vi "test1-ProcessSyncMessageInCSMLoop(OnlyReceive).vi"(8 "error in (no error)":errorcluster, 11 "TestCase in":refnum<class "testcase-CSMAddonLoopSupport.lvclass">) -> (0 "error out":errorcluster, 3 "TestCase out":refnum<class "testcase-CSMAddonLoopSupport.lvclass">)   [LabVIEW 2017, in "testcase-CSMAddonLoopSupport.lvclass"]
uses:
  testcase-CSMAddonLoopSupport.lvclass
  4585ddd5-ba69-4fd4-94fe-207595864cbd.vi
  a7620e19-6451-46a1-85ca-ade5edb58587.vi
  55fec5d7-cd22-46f7-b641-2c7c49619fc8.vi
  <vilib>/addons/_JKI Toolkits/VI Tester/TestCase.llb/TestCase.lvclass
  src/user.lib/_NEVSTOP/Communicable State Machine(CSM)/Communicable State Machine.lvlib
  C:/Program Files (x86)/National Instruments/LabVIEW 2017/vi.lib/addons/_JKI Toolkits/VI Tester/TestCase.llb/TestCase.lvclass
panel:
  out "error out2":errorcluster
  out "LoopCount":i32
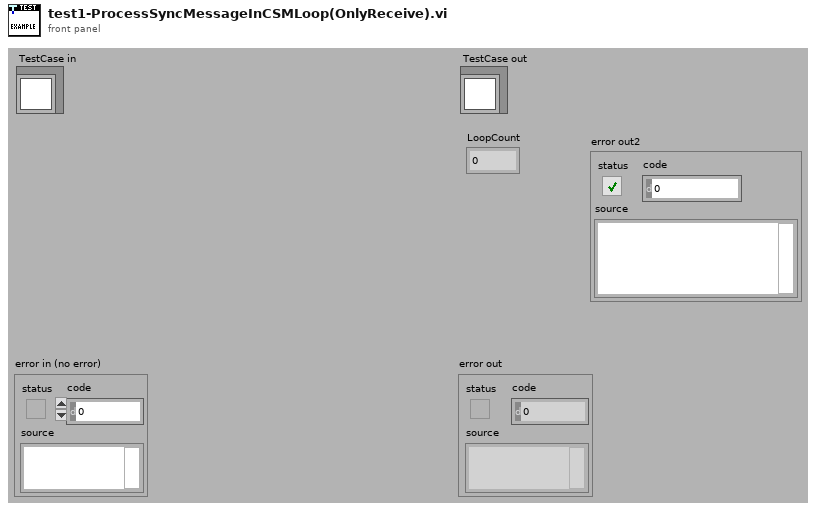
[diagram p1: front panel]
types:
  T1 = cluster{"Arguments":string, "Response":string, "error":errorcluster}
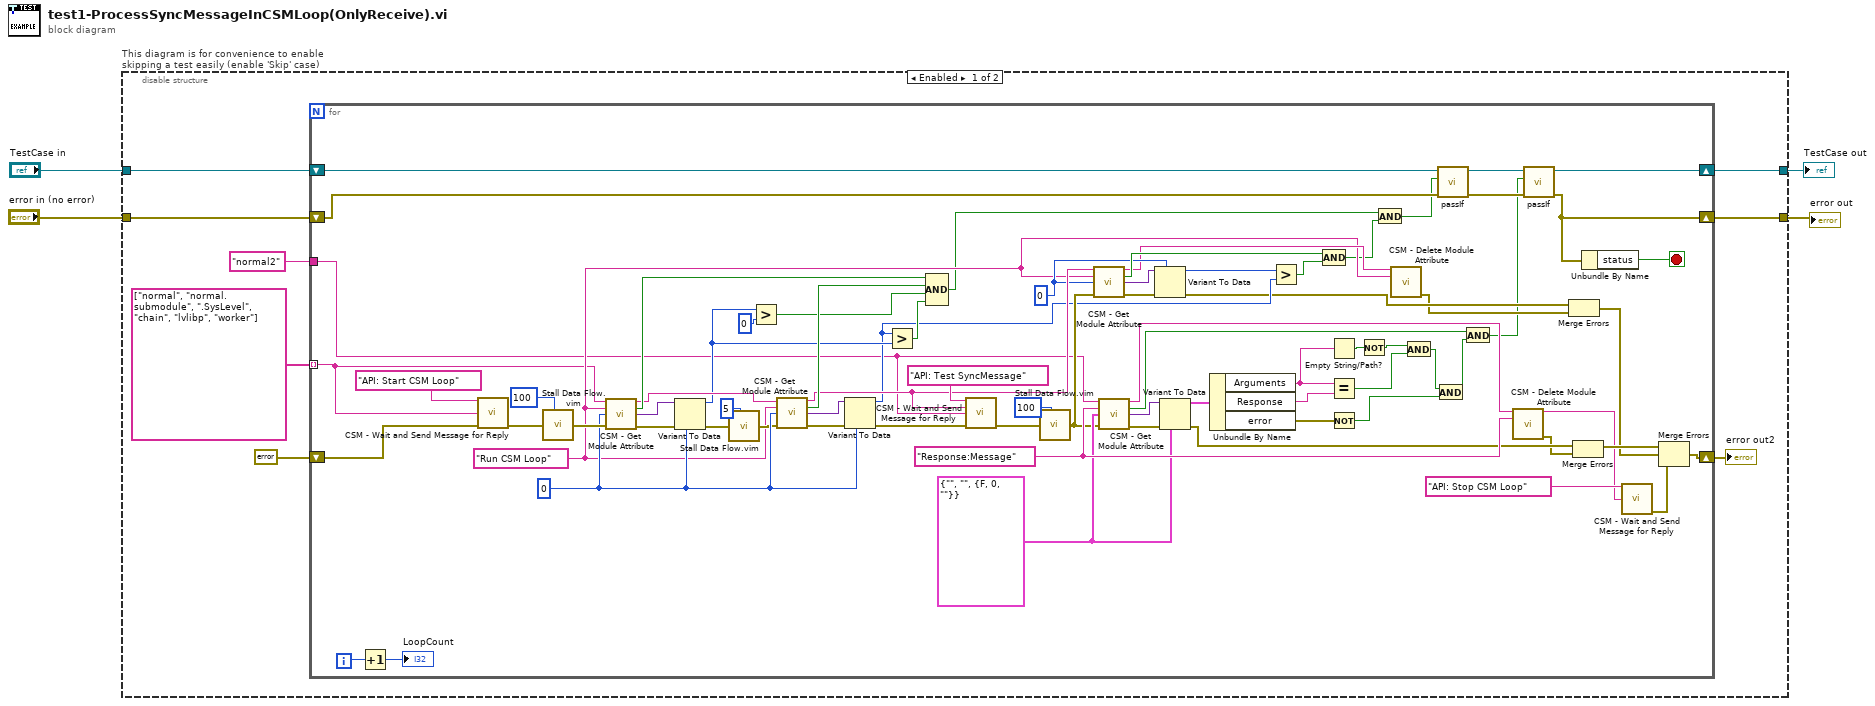
[diagram p0: block diagram]
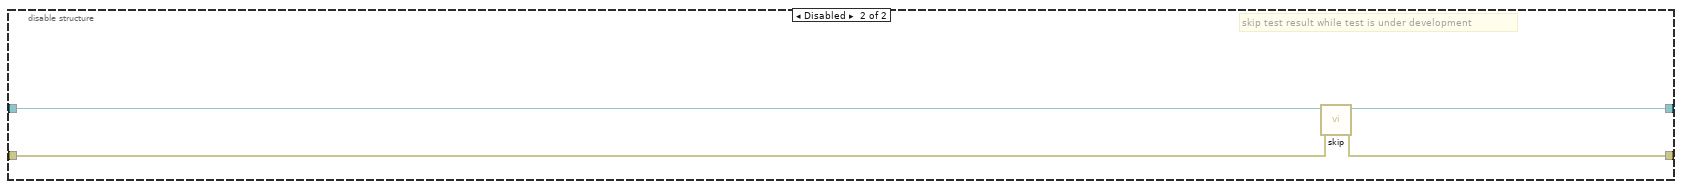
[diagram p2: hidden frame]
diagram:
  n1 = disable-structure "This diagram is for convenience to enable skipping a test easily (enable 'Skip' case)" shown="Enabled" {
    disable-tunnel: "TestCase in" -> [w11 w92]
    disable-tunnel: [w9 w90] -> w1
    disable-tunnel: [w8 w91] -> w3
    disable-tunnel: "error in (no error)" -> [w10 w89]
    frame Enabled {
      n2 = for {
        tunnel: string[] ["normal", "normal.submodule", ".SysLevel", "chain", "lvlibp", "worker"] -> [w16] mode=indexing
        shift-right: [w21] -> w9
        shift-left: w11 -> [w28]
        shift-right: [w20] -> w8
        shift-left: w10 -> [w27]
        tunnel: "normal2" ("CSM") -> [w13]
        shift-right: [w29] -> w5
        shift-left: errorcluster {"status"=FALSE, "code"=0, "source"=""} ("error in (no error)") -> [w83]
        i -> [w88]
        stop <- w19 stop-if-true
        w38 = u32 0
        w53 = u32 0
        w34 = "Run CSM Loop" ("State")
        w64 = T1 {"Arguments"="", "Response"="", "error"={"status"=FALSE, "code"=0, "source"=""}}
        w65 = "Response:Message" ("State")
        n3 = Increment(x=w88) -> (x+1=→"LoopCount":i32)
        n4 = call "CSM - Wait and Send Message for Reply.vi"("State"="API: Start CSM Loop", "Target Module"=w16, "Error In (No Error)"=w83) -> ("error out"=w85:errorcluster)  [unwired: 9 in, 3 out]
        n5 = call "Stall Data Flow.vim"("value in"=w85, "milliseconds to wait"=u32 100) -> ("value out"=w61:errorcluster)  [unwired: 1 out]
        n6 = call "CSM - Get Module Attribute.vi"("CSM Name"=w16, "Attribute"=w34, "Default Value (Empty Variant)"=w53, "Error In"=w61) -> ("CSM Name (Dup)"=w55:string, "Found"=w60:bool, "Value"=w54:variant, "error out"=w58:errorcluster)  [unwired: 7 in, 1 out]
        n7 = Variant To Data(error in=w58, type=w53, Variant=w54) -> (data=w48:u32, error out=w47:errorcluster)
        n8 = call "Stall Data Flow.vim"("value in"=w47, "milliseconds to wait"=u32 5) -> ("value out"=w46:errorcluster)  [unwired: 1 out]
        n9 = Greater?(x=w48, y=u32 0) -> (0:w51:bool)
        n10 = call "CSM - Get Module Attribute.vi"("CSM Name"=w55, "Attribute"=w34, "Default Value (Empty Variant)"=w53, "Error In"=w46) -> ("CSM Name (Dup)"=w43:string, "Found"=w59:bool, "Value"=w50:variant, "error out"=w57:errorcluster)  [unwired: 7 in, 1 out]
        n11 = Variant To Data(error in=w57, type=w53, Variant=w50) -> (data=w36:u32, error out=w56:errorcluster)
        n12 = Greater?(x=w36, y=w48) -> (0:w49:bool)
        n13 = Compound Arithmetic op=AND(w60, w59, w51, w49) -> (w26:bool)
        n14 = call "CSM - Wait and Send Message for Reply.vi"("State"="API: Test SyncMessage", "Arguments (\"\")"=w43, "Target Module"=w13, "Error In (No Error)"=w56) -> ("error out"=w80:errorcluster)  [unwired: 8 in, 3 out]
        n15 = call "Stall Data Flow.vim"("value in"=w80, "milliseconds to wait"=u32 100) -> ("value out"=w44:errorcluster)  [unwired: 1 out]
        n16 = call "CSM - Get Module Attribute.vi"("CSM Name"=w43, "Attribute"=w34, "Default Value (Empty Variant)"=w38, "Error In"=w44) -> ("CSM Name (Dup)"=w35:string, "Found"=w40:bool, "Value"=w39:variant, "error out"=w41:errorcluster)  [unwired: 7 in, 1 out]
        n17 = call "CSM - Get Module Attribute.vi"("CSM Name"=w13, "Attribute"=w65, "Default Value (Empty Variant)"=w64, "Error In"=w44) -> ("CSM Name (Dup)"=w73:string, "Found"=w75:bool, "Value"=w78:variant, "error out"=w79:errorcluster)  [unwired: 7 in, 1 out]
        n18 = Variant To Data(error in=w41, type=w38, Variant=w39) -> (data=w37:u32, error out=w33:errorcluster)
        n19 = Variant To Data(error in=w79, type=w64, Variant=w78) -> (data=w77:T1, error out=w63:errorcluster)
        n20 = Unbundle By Name(w77) -> ("Arguments"=w68:string, "Response"=w67:string, "error"=w66:errorcluster)
        n21 = Greater?(x=w37, y=w36) -> (0:w42:bool)
        n22 = Compound Arithmetic op=AND(w40, w42) -> (w25:bool)
        n23 = Empty String/Path?(string/path=w68) -> (empty?=w72:bool)
        n24 = Equal?(x=w68, y=w67) -> (x = y?=w70:bool)
        n25 = Not(x=w66) -> (.not. x?=w76:bool)
        n26 = Not(x=w72) -> (.not. x?=w71:bool)
        n27 = And(x=w26, y=w25) -> (x .and. y?=w24:bool)
        n28 = call "CSM - Delete Module Attribute.vi"("CSM Name"=w35, "Attribute"=w34) -> ("error out"=w32:errorcluster)  [unwired: 10 in, 3 out]
        n29 = And(x=w71, y=w70) -> (x .and. y?=w69:bool)
        n30 = And(x=w69, y=w76) -> (x .and. y?=w74:bool)
        n31 = call-dynamic "passIf.vi"("error in (no error)"=w27, "pass"=w24, "TestCase in"=w28) -> ("error out"=w22:errorcluster, "TestCase out"=w23:refnum<class "testcase-CSMAddonLoopSupport.lvclass">)  [unwired: 7 in]
        n32 = And(x=w75, y=w74) -> (x .and. y?=w18:bool)
        n33 = call "CSM - Delete Module Attribute.vi"("CSM Name"=w73, "Attribute"=w65) -> ("CSM Name (Dup)"=w15:string, "error out"=w62:errorcluster)  [unwired: 10 in, 2 out]
        n34 = call-dynamic "passIf.vi"("error in (no error)"=w22, "pass"=w18, "TestCase in"=w23) -> ("error out"=w20:errorcluster, "TestCase out"=w21:refnum<class "testcase-CSMAddonLoopSupport.lvclass">)  [unwired: 7 in]
        n35 = Merge Errors(w33, w32) -> (w30:errorcluster)
        n36 = Merge Errors(w63, w62) -> (w31:errorcluster)
        n37 = Unbundle By Name(w20) -> ("status"=w19:bool)
        n38 = call "CSM - Wait and Send Message for Reply.vi"("State"="API: Stop CSM Loop", "Target Module"=w15) -> ("error out"=w14:errorcluster)  [unwired: 10 in, 3 out]
        n39 = Merge Errors(w31, w30, w14) -> (w29:errorcluster)
      }
      "error out2" <- w5
    }
    frame Disabled {
      # "skip test result while test is under development"
      n40 = call <vilib>:"skip.vi"("error in (no error)"=w89, "TestCase in"=w92) -> ("error out"=w91:errorcluster, "TestCase out"=w90:refnum<class "testcase-CSMAddonLoopSupport.lvclass">)  [unwired: 8 in]
    }
  }
  "error out" <- w3
  "TestCase out" <- w1
